vi "DLLHandler.vi"(0 "connection ID":i32, 5 "results_cluster":refnum<vi>[](array[refnum]), 7 "params_cluster":refnum<vi>[](array[refnum]), 9 "method":string, 11 "error":errorcluster) -> (4 "connection ID out":i32, 15 "error":errorcluster)   [LabVIEW 2016]
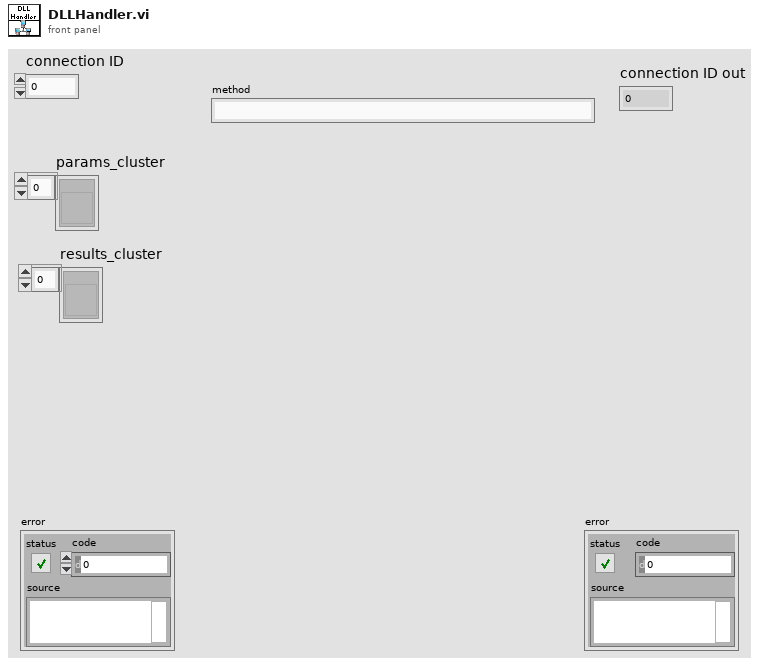
[diagram p1: front panel]
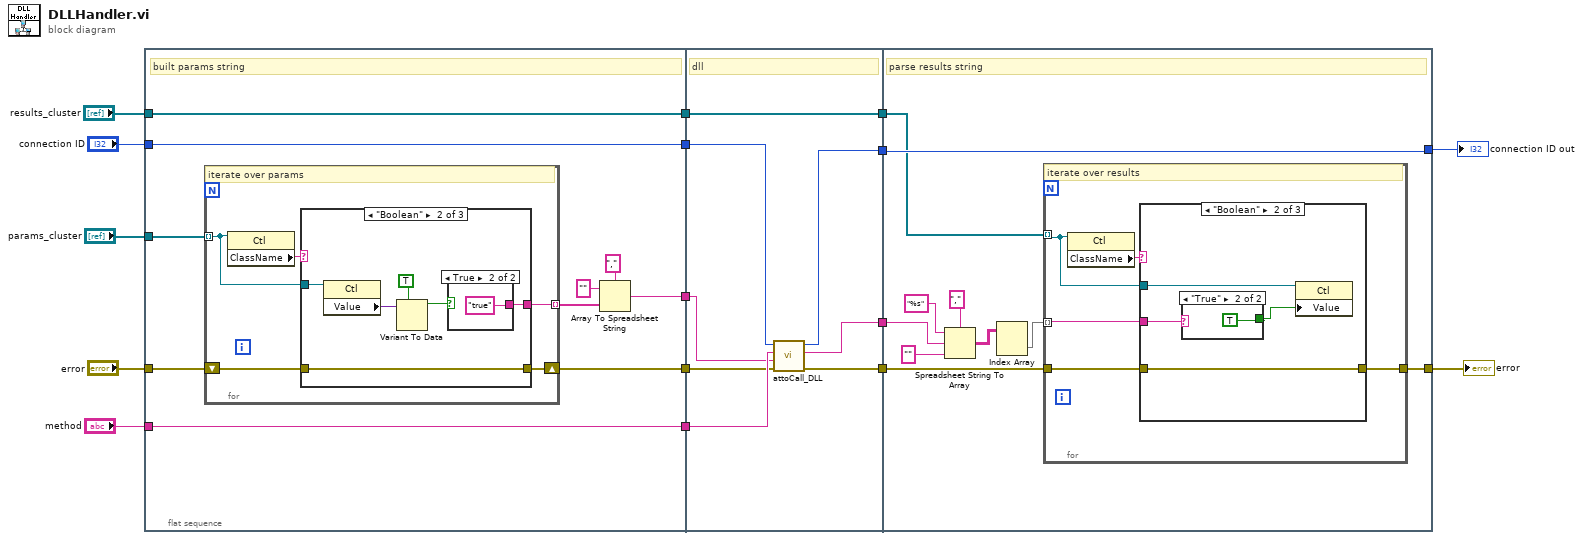
[diagram p0: block diagram]
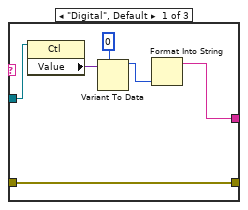
[diagram p2: hidden frame]
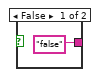
[diagram p3: hidden frame]
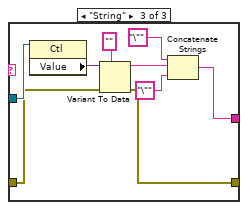
[diagram p4: hidden frame]
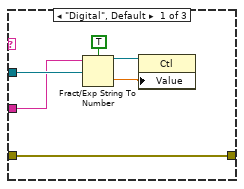
[diagram p5: hidden frame]
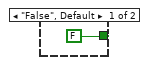
[diagram p6: hidden frame]
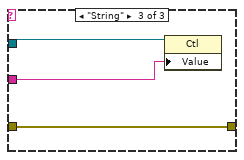
[diagram p7: hidden frame]
diagram:
  n1 = flat-sequence {
    tunnel: "error" -> [w19]
    tunnel: "connection ID" -> [w26]
    tunnel: [w26] -> w16
    tunnel: [w18] -> w15
    tunnel: "method" -> [w20]
    tunnel: "params_cluster" -> [w22]
    tunnel: "results_cluster" -> [w21]
    tunnel: [w21] -> w6
    tunnel: [w20] -> w4
    tunnel: [w17] -> w1
    tunnel: w16 -> [w62]
    tunnel: w15 -> [w56]
    tunnel: [w61] -> w11
    tunnel: [w60] -> w10
    tunnel: [w59] -> w9
    tunnel: w6 -> [w58]
    tunnel: [w58] -> w5
    tunnel: w4 -> [w57]
    tunnel: w1 -> [w55]
    tunnel: [w70] -> w8
    tunnel: [w72] -> w2
    tunnel: w11 -> [w72]
    tunnel: w10 -> [w66]
    tunnel: w9 -> [w71]
    tunnel: w5 -> [w69]
    frame #0 {
      # "built params string"
      n2 = for {
        tunnel: w22 -> [w30] mode=indexing
        tunnel: [w29] -> w25 mode=indexing
        shift-right: [w27] -> w18
        shift-left: w19 -> [w28]
        # "iterate over params"
        n3 = property class="Ctl"(reference=w30) -> ("ClassName"=w31:string)  [unwired: 1 in, 2 out]
        n4 = case shown="\"Boolean\"" w31 {
          tunnel: w30 -> [w37 w43 w54]
          tunnel: [w33 w39 w50] -> w29
          tunnel: w28 -> [w32 w38 w47]
          tunnel: [w32 w38 w46] -> w27
          frame "Digital", Default {
            n5 = property class="Ctl"(reference=w37) -> ("Value"=w35:variant)  [unwired: 1 in, 2 out]
            n6 = Variant To Data(type=0, Variant=w35) -> (data=w34:i32)  [unwired: 1 in, 1 out]
            n7 = Format Into String(w34) -> (resulting string=w33:string)  [unwired: 3 in, 1 out]
          }
          frame "Boolean" {
            n8 = property class="Ctl"(reference=w43) -> ("Value"=w41:variant)  [unwired: 1 in, 2 out]
            n9 = Variant To Data(type=TRUE, Variant=w41) -> (data=w40:bool)  [unwired: 1 in, 1 out]
            n10 = case shown="True" w40 {
              tunnel: ["false" "true"] -> w39
              frame False {
              }
              frame True {
              }
            }
          }
          frame "String" {
            n11 = property class="Ctl"(reference=w54) -> ("Value"=w53:variant)  [unwired: 1 in, 2 out]
            n12 = Variant To Data(error in=w47, type="", Variant=w53) -> (data=w51:string, error out=w46:errorcluster)
            n13 = Concatenate Strings("\"" ("string"), w51, "\"" ("string")) -> (w50:string)
          }
        }
      }
      n14 = Array To Spreadsheet String(delimiter (Tab)=",", array=w25, 3:"" ("format string")) -> (spreadsheet string=w17:string)
    }
    frame #1 {
      # "dll"
      n15 = call "attoCall_DLL.vi"("error in"=w56, "params"=w55, "method"=w57, "deviceHandle"=w62) -> ("error out"=w59:errorcluster, "response"=w60:string, "deviceHandle out"=w61:i32)  [unwired: 5 in]
    }
    frame #2 {
      # "parse results string"
      n16 = Spreadsheet String To Array(delimiter (Tab)=",", format string="%s", spreadsheet string=w66, array type (2D Dbl)="" ("format string")) -> (array=w64:string[][])
      n17 = Index Array(array=w64) -> (element=w63:string[])  [unwired: 2 in]
      n18 = for {
        tunnel: w63 -> [w77] mode=indexing
        tunnel: w69 -> [w75] mode=indexing
        tunnel: [w74] -> w70
        tunnel: w71 -> [w73]
        # "iterate over results"
        n19 = property class="Ctl"(reference=w75) -> ("ClassName"=w76:string)  [unwired: 1 in, 2 out]
        n20 = case shown="\"Boolean\"" w76 {
          tunnel: w77 -> [w81 w83 w89]
          tunnel: w75 -> [w82 w86 w91]
          tunnel: [w78 w85 w90] -> w74
          tunnel: w73 -> [w78 w85 w90]
          frame "Digital", Default {
            n21 = Fract/Exp String To Number(use system decimal point (T)=TRUE, string=w81) -> (number=w80:dbl)  [unwired: 2 in, 1 out]
            n22 = property class="Ctl"(reference=w82, "Value"=w80) -> ()  [unwired: 1 in, 2 out]
          }
          frame "Boolean" {
            n23 = case shown="\"True\"" w83 {
              tunnel: [FALSE TRUE] -> w84
              frame "False", Default {
              }
              frame "True" {
              }
            }
            n24 = property class="Ctl"(reference=w86, "Value"=w84) -> ()  [unwired: 1 in, 2 out]
          }
          frame "String" {
            n25 = property class="Ctl"(reference=w91, "Value"=w89) -> ()  [unwired: 1 in, 2 out]
          }
        }
      }
    }
  }
  "error" <- w8
  "connection ID out" <- w2
